vi "Sort and Filter SysLog History.vi"(6 "Spaltenindex intern":u32, 7 "NoSort":bool, 8 "Fehler (in)":errorcluster caption="Fehlerkonstante", 10 "Cluster (in)":T1, 11 "Array-Typ (2D Dbl) in":string[][](array[string])) -> (0 "Fehler (out)":errorcluster caption="Fehlerkonstante", 3 "Array-Typ (2D Dbl) out":string[][](array[string]))   [LabVIEW 2015, in "SysLog.lvlib"]
doc: "Spaltenindex intern:\n1 ... wenn PC/cRIO aus LogFile laden bereits vorhanden,\n0 ... für Systusanzeige\nNoSort:\nTRUE ...für Statusanzeige notwendig (selbe Reihenfolge wie Symbole)\nFALSE ... für LogFile/Viewer"
uses:
  SysLog.lvlib
  SysLogSort.ctl
  Allgemein/allgemeine Sub-VIs.lvlib
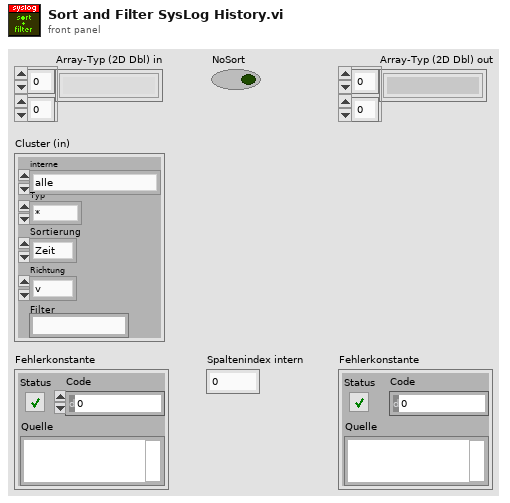
[diagram p1: front panel]
types:
  T1 = typedef "SysLog.lvlib/SysLogSort.ctl" = cluster{"interne":enum16{"alle", "nur benutzerrelevante", "nur interne"}, "Typ":enum16{"*", "Err+Warn", "Err", "Warn", "OK"}, "Sortierung":enum16{"Zeit", "Code", "Typ"}, "Richtung":enum16{"v", "^"}, "Filter":string}
  T2 = cluster{"Index der Spalte des Sortierschlüssels (0)":i32, "Suchspalte besteht aus Zahlen (F)":bool}
  T3 = enum16{"alle", "nur benutzerrelevante", "nur interne"}
  T4 = cluster{"Index der Spalte des Sortierschlüssels (0)":i32, "Filter":string, "Aktion":enum16{"entfernen", "nur diese belassen"}}
  T5 = cluster{"Spaltenindex intern":u32, string[], "Aktion":enum16{"entfernen", "nur diese belassen"}}
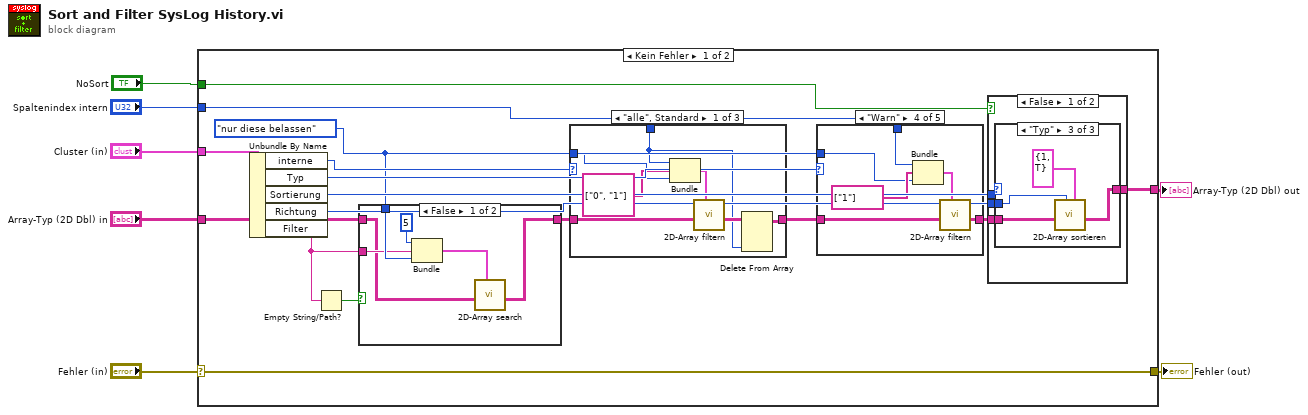
[diagram p0: block diagram]
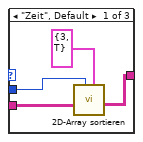
[diagram p3: hidden frame]
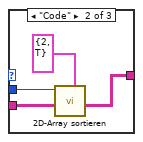
[diagram p4: hidden frame]
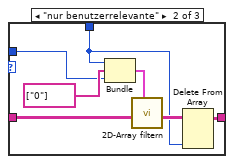
[diagram p6: hidden frame]
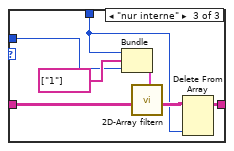
[diagram p7: hidden frame]
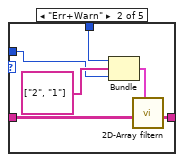
[diagram p9: hidden frame]
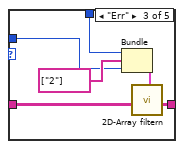
[diagram p10: hidden frame]
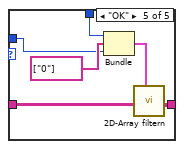
[diagram p11: hidden frame]
diagram:
  n1 = case shown="Kein Fehler" "Fehler (in)" {
    selector: "Fehler (in)" -> [w23 w95]
    tunnel: [w23 w95] -> w6
    tunnel: "Cluster (in)" -> [w22 _]
    tunnel: "Array-Typ (2D Dbl) in" -> [w11 w94]
    tunnel: [w20 w94] -> w3
    tunnel: "Spaltenindex intern" -> [w14 _]
    tunnel: "NoSort" -> [w13 _]
    frame No Error {
      w9 = enum16{"entfernen", "nur diese belassen"}."nur diese belassen" ("Aktion")
      n2 = Unbundle By Name(w22) -> ("interne"=w16:T3, "Typ"=w18:enum16{"*", "Err+Warn", "Err", "Warn", "OK"}, "Sortierung"=w21:enum16{"Zeit", "Code", "Typ"}, "Richtung"=w19:enum16{"v", "^"}, "Filter"=w8:string)
      n3 = Empty String/Path?(string/path=w8) -> (empty?=w12:bool)
      n4 = case shown="False" w12 {
        tunnel: w11 -> [w25 w30]
        tunnel: [w24 w30] -> w10
        tunnel: w9 -> [w29 _]
        tunnel: w8 -> [w27 _]
        frame False {
          n5 = Bundle("Index der Spalte des Sortierschlüssels (0)"=5, "Filter"=w27, "Aktion"=w29) -> (w26:T4)  [unwired: 1 in]
          n6 = call "2D-Array search.vi"("Cluster"=w26, "2D-String-Array_in"=w25) -> ("2D-String-Array_gefiltert"=w24:string[][])  [unwired: 9 in]
        }
        frame True {
        }
      }
      n7 = case shown="\"alle\", Standard" w16 {
        tunnel: w10 -> [w54 w61 w68]
        tunnel: [w49 w56 w63] -> w15
        tunnel: w9 -> [w51 w59 w66]
        tunnel: w14 -> [w48 w55 w62]
        frame "alle", Default {
          n8 = Bundle("Spaltenindex intern"=w48, string[] ["0", "1"], "Aktion"=w51) -> (w53:T5)  [unwired: 1 in]
          n9 = call "2D-Array filtern.vi"("Cluster"=w53, "2D-String-Array_in"=w54) -> ("2D-String-Array_gefiltert"=w50:string[][])  [unwired: 9 in]
          n10 = Delete From Array(array=w50, index (col)=w48) -> (array with subset deleted=w49:string[][])  [unwired: 2 in, 1 out]
        }
        frame "nur benutzerrelevante" {
          n11 = Bundle("Spaltenindex intern"=w55, string[] ["0"], "Aktion"=w59) -> (w58:T5)  [unwired: 1 in]
          n12 = call "2D-Array filtern.vi"("Cluster"=w58, "2D-String-Array_in"=w61) -> ("2D-String-Array_gefiltert"=w57:string[][])  [unwired: 9 in]
          n13 = Delete From Array(array=w57, index (col)=w55) -> (array with subset deleted=w56:string[][])  [unwired: 2 in, 1 out]
        }
        frame "nur interne" {
          n14 = Bundle("Spaltenindex intern"=w62, string[] ["1"], "Aktion"=w66) -> (w65:T5)  [unwired: 1 in]
          n15 = call "2D-Array filtern.vi"("Cluster"=w65, "2D-String-Array_in"=w68) -> ("2D-String-Array_gefiltert"=w64:string[][])  [unwired: 9 in]
          n16 = Delete From Array(array=w64, index (col)=w62) -> (array with subset deleted=w63:string[][])  [unwired: 2 in, 1 out]
        }
      }
      n17 = case shown="\"Warn\"" w18 {
        tunnel: w15 -> [w69 w75 w81 w87 w93]
        tunnel: [w69 w74 w80 w86 w92] -> w17
        tunnel: w9 -> [_ w71 w78 w84 w89]
        tunnel: w14 -> [_ w70 w76 w82 w88]
        frame "*", Default {
        }
        frame "Err+Warn" {
          n18 = Bundle("Spaltenindex intern"=w70, string[] ["2", "1"], "Aktion"=w71) -> (w73:T5)  [unwired: 1 in]
          n19 = call "2D-Array filtern.vi"("Cluster"=w73, "2D-String-Array_in"=w75) -> ("2D-String-Array_gefiltert"=w74:string[][])  [unwired: 9 in]
        }
        frame "Err" {
          n20 = Bundle("Spaltenindex intern"=w76, string[] ["2"], "Aktion"=w78) -> (w77:T5)  [unwired: 1 in]
          n21 = call "2D-Array filtern.vi"("Cluster"=w77, "2D-String-Array_in"=w81) -> ("2D-String-Array_gefiltert"=w80:string[][])  [unwired: 9 in]
        }
        frame "Warn" {
          n22 = Bundle("Spaltenindex intern"=w82, string[] ["1"], "Aktion"=w84) -> (w83:T5)  [unwired: 1 in]
          n23 = call "2D-Array filtern.vi"("Cluster"=w83, "2D-String-Array_in"=w87) -> ("2D-String-Array_gefiltert"=w86:string[][])  [unwired: 9 in]
        }
        frame "OK" {
          n24 = Bundle("Spaltenindex intern"=w88, string[] ["0"], "Aktion"=w89) -> (w90:T5)  [unwired: 1 in]
          n25 = call "2D-Array filtern.vi"("Cluster"=w90, "2D-String-Array_in"=w93) -> ("2D-String-Array_gefiltert"=w92:string[][])  [unwired: 9 in]
        }
      }
      n26 = case shown="False" w13 {
        tunnel: w21 -> [w34 _]
        tunnel: [w33 w47] -> w20
        tunnel: w19 -> [w32 _]
        tunnel: w17 -> [w31 w47]
        frame False {
          n27 = case shown="\"Typ\"" w34 {
            tunnel: [w38 w42 w43] -> w33
            tunnel: w32 -> [w36 w40 w44]
            tunnel: w31 -> [w35 w39 w45]
            frame "Zeit", Default {
              n28 = call "2D-Array sortieren.vi"("Suchvorgabe"=T2 {"Index der Spalte des Sortierschlüssels (0)"=3, "Suchspalte besteht aus Zahlen (F)"=TRUE}, "Richtung"=w36, "2D-String-Array_in"=w35) -> ("2D-String-Array_nach Spalte 0 sortiert"=w38:string[][])  [unwired: 8 in]
            }
            frame "Code" {
              n29 = call "2D-Array sortieren.vi"("Suchvorgabe"=T2 {"Index der Spalte des Sortierschlüssels (0)"=2, "Suchspalte besteht aus Zahlen (F)"=TRUE}, "Richtung"=w40, "2D-String-Array_in"=w39) -> ("2D-String-Array_nach Spalte 0 sortiert"=w42:string[][])  [unwired: 8 in]
            }
            frame "Typ" {
              n30 = call "2D-Array sortieren.vi"("Suchvorgabe"=T2 {"Index der Spalte des Sortierschlüssels (0)"=1, "Suchspalte besteht aus Zahlen (F)"=TRUE}, "Richtung"=w44, "2D-String-Array_in"=w45) -> ("2D-String-Array_nach Spalte 0 sortiert"=w43:string[][])  [unwired: 8 in]
            }
          }
        }
        frame True {
        }
      }
    }
    frame Error {
    }
  }
  "Fehler (out)" <- w6
  "Array-Typ (2D Dbl) out" <- w3
